vi "Set_Rate.vi"(8 "error in (no error)":errorcluster, 10 "Frequency":dbl[unit], 11 "Thorlabs_PM100D in":refnum<class "Thorlabs_PM100D.lvclass">) -> (0 "error out":errorcluster, 3 "Thorlabs_PM100D out":refnum<class "Thorlabs_PM100D.lvclass">)   [LabVIEW 2020, in "Thorlabs_PM100D.lvclass"]
uses:
  <instrlib>/Classes/Powermeter/Thorlabs_PM100D/Thorlabs_PM100D.lvclass
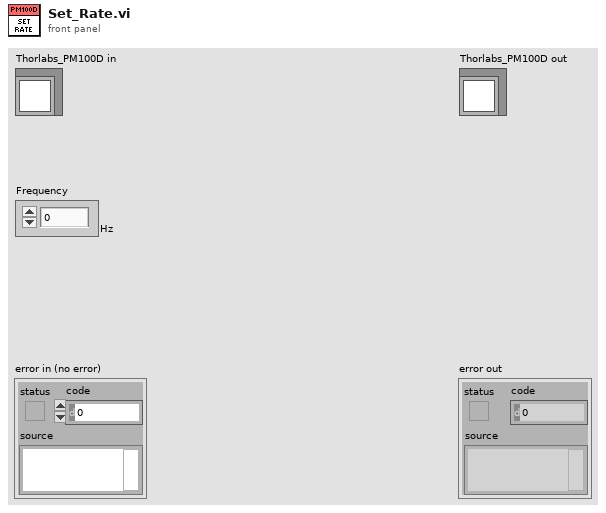
[diagram p1: front panel]
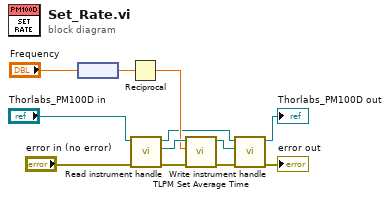
[diagram p0: block diagram]
diagram:
  n1 = node("Frequency") -> (w9:dbl)
  n2 = Reciprocal(x=w9) -> (1/x=w8:dbl)
  n3 = call-dynamic "Read instrument handle.vi"("error in (no error)"="error in (no error)", "Thorlabs_PM100D in"="Thorlabs_PM100D in") -> ("error out"=w7:errorcluster, "instrument handle"=w11:refnum<visa-resource-name>, "Thorlabs_PM100D out"=w5:refnum<class "Thorlabs_PM100D.lvclass">)  [unwired: 7 in]
  n4 = call <instrlib>:"TLPM Set Average Time.vi"("error in (no error)"=w7, "Average Time (0.0)"=w8, "instrument handle"=w11) -> ("error out"=w3:errorcluster, "instrument handle out"=w4:refnum<visa-resource-name>)  [unwired: 7 in]
  n5 = call-dynamic "Write instrument handle.vi"("error in (no error)"=w3, "instrument handle"=w4, "Thorlabs_PM100D in"=w5) -> ("error out"=→"error out":errorcluster, "Thorlabs_PM100D out"=→"Thorlabs_PM100D out":refnum<class "Thorlabs_PM100D.lvclass">)  [unwired: 7 in]
